vi "logSelection.vi"(2 "Controls[]":refnum<vi>[](array[refnum]), 3 "log_from":string) -> (0 "cluster_out":cluster{"Label.Text":string, bool}[](array[cluster]), 1 "log_from out":string)   [LabVIEW 2021]
panel:
  in  "stop":bool
  in  "cluster_select":cluster{"Label.Text":string, bool}[](array[cluster])
  # "Index"
  # "Log from:"
  # "ELEMENTS TO LOG:\n\n1. Select the elements you want to log by \n     pressing the round button on each element.\n\n2. Navigate the cluster using the Index.\n    Ensure you have discovered all elements.\n\n3. Once you have finished push the OK button."
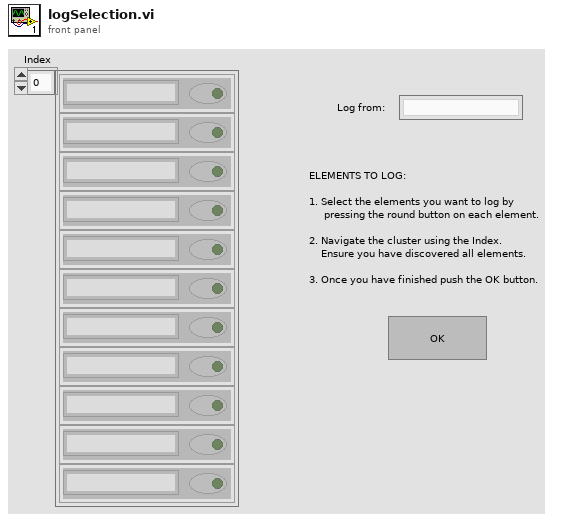
[diagram p1: front panel]
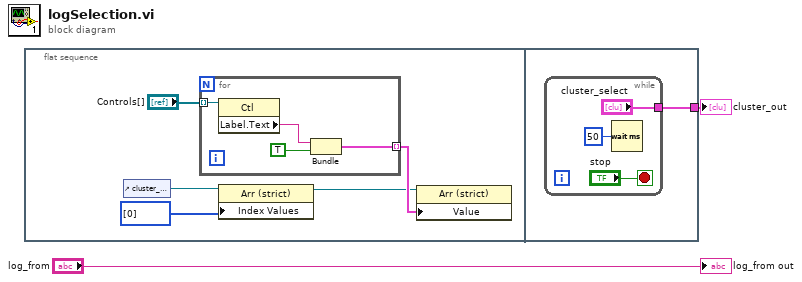
[diagram p0: block diagram]
diagram:
  n1 = flat-sequence {
    tunnel: [w12] -> w2
    frame #0 {
      n2 = control-ref of="cluster_select"() -> (w4:refnum<vi>)
      n3 = for {
        tunnel: "Controls[]" -> [w9] mode=indexing
        tunnel: [w10] -> w6 mode=indexing
        n4 = property class="Ctl"(reference=w9) -> ("Label.Text"=w8:string)  [unwired: 1 in, 2 out]
        n5 = Bundle("Label.Text"=w8, TRUE) -> (w10:cluster{"Label.Text":string, bool})  [unwired: 1 in]
      }
      n6 = property class="Arr (strict)"(reference=w4, "Index Values"=u32[] [0]) -> (reference out=w3:refnum<vi>)  [unwired: 1 in, 1 out]
      n7 = property class="Arr (strict)"(reference=w3, "Value"=w6) -> ()  [unwired: 1 in, 2 out]
    }
    frame #1 {
      n8 = while {
        tunnel: ["cluster_select"] -> w12
        stop <- "stop" stop-if-true
        n9 = Wait (ms)(milliseconds to wait=u32 50) -> ()  [unwired: 1 out]
      }
    }
  }
  "cluster_out" <- w2
  "log_from out" <- "log_from"
